vi "test_sampling.vi"() -> ()   [LabVIEW 2017]
uses:
  <vilib>/Analysis/2dsp.llb/1D Convolution (DBL).vi
  <vilib>/Analysis/NI_AALBase.lvlib
  <vilib>/Analysis/NI_AALPro.lvlib
panel:
  out "32비트 정수":i32
  out "FFT signal 3":waveform(dbl)(graph)
  out "FFT signal 2":waveform(dbl)(graph)
  out "크기 2":i32
  out "signal 2":waveform(dbl)(graph)
  in  "sampling time(sec)":dbl=0.5
  out "크기":i32
  out "Array":dbl[](array[numeric])
  out "FFT signal":waveform(dbl)(graph)
  out "signal":waveform(dbl)(graph)
  in  "Frequency(Hz)":dbl=614000.0
  in  "Amplitude(Vpeak)":dbl=1.0
  in  "Pulse length(sec)":dbl=0.5
  in  "Sampling frequency(Hz)":dbl=3000000.0
  in  "Delay time.A.1(sec)":dbl=0.5
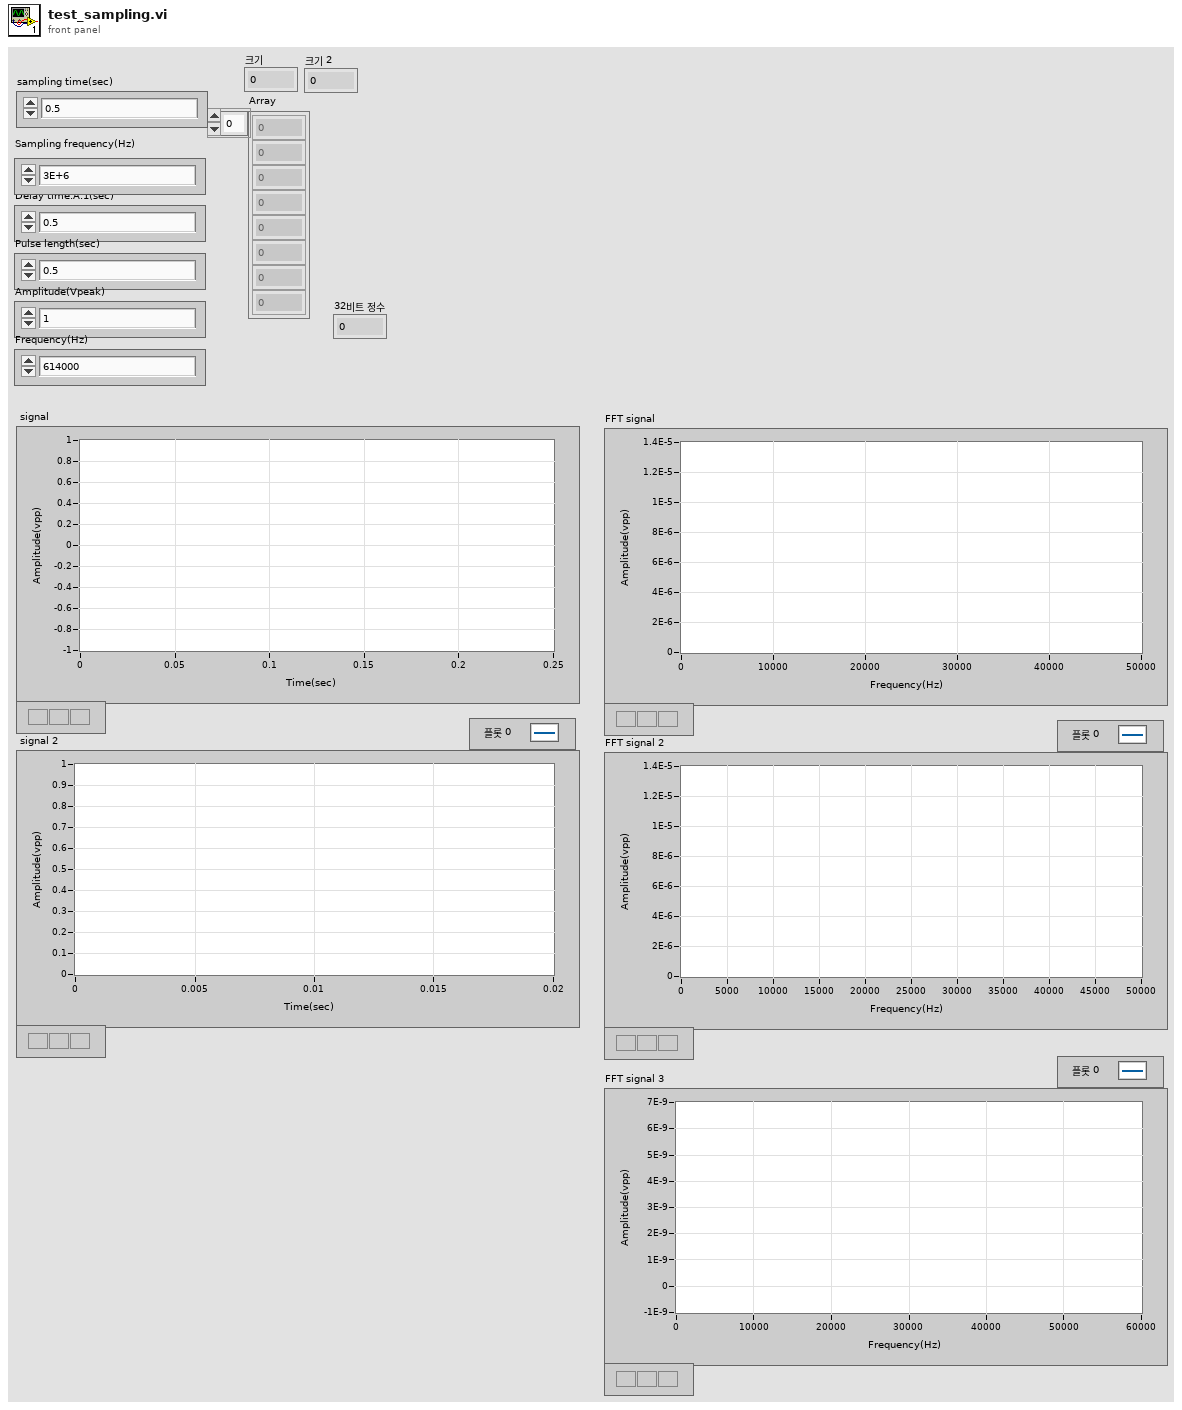
[diagram p1: front panel]
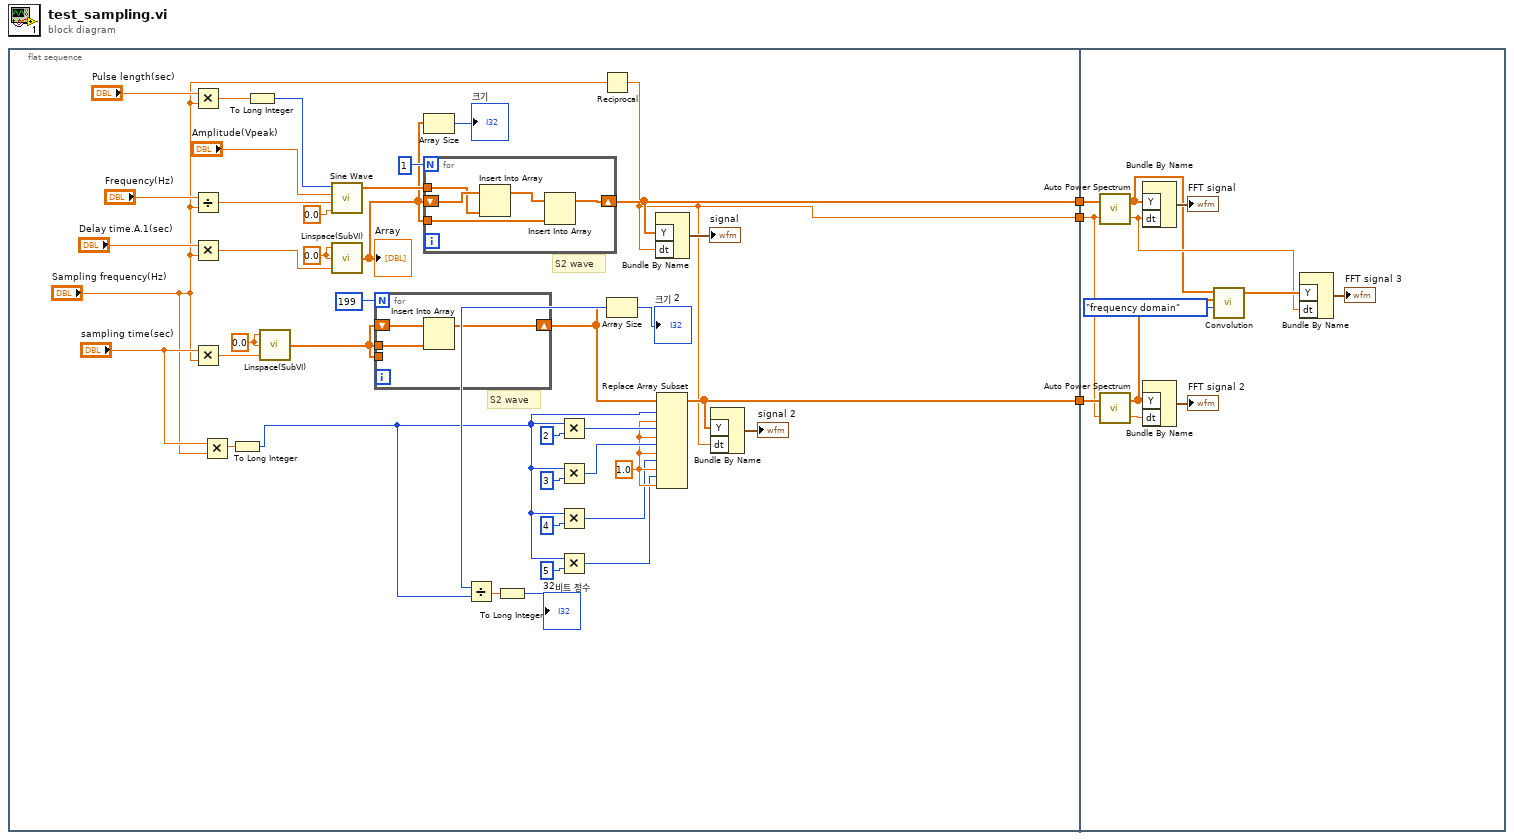
[diagram p0: block diagram]
diagram:
  n1 = flat-sequence {
    tunnel: [w30] -> w3
    tunnel: [w5] -> w2
    tunnel: [w19] -> w1
    tunnel: w3 -> [w63]
    tunnel: w2 -> [w58]
    tunnel: w1 -> [w59]
    frame #0 {
      w18 = 1.0 ("새 원소/부분배열")
      w27 = 0.0 ("Start")
      w36 = 0.0 ("Start")
      # "S2 wave"
      # "S2 wave"
      n2 = Multiply(x="Pulse length(sec)", y="Sampling frequency(Hz)") -> (x*y=w42:dbl)
      n3 = Divide(x="Frequency(Hz)", y="Sampling frequency(Hz)") -> (x/y=w38:dbl)
      n4 = Multiply(x="Delay time.A.1(sec)", y="Sampling frequency(Hz)") -> (x*y=w34:dbl)
      n5 = Multiply(x="sampling time(sec)", y="Sampling frequency(Hz)") -> (x*y=w26:dbl)
      n6 = Multiply(x="sampling time(sec)", y="Sampling frequency(Hz)") -> (x*y=w11:dbl)
      n7 = To Long Integer(number=w11) -> (32bit integer=w9:i32)
      n8 = To Long Integer(number=w42) -> (32bit integer=w41:i32)
      n9 = call "Linspace(SubVI).vi"("NumElements"=w26, "End"=w27, "Start"=w27) -> ("Array"=w7:dbl[])
      n10 = call <vilib>:"Sine Wave.vi"("samples"=w41, "amplitude"="Amplitude(Vpeak)", "frequency"=w38, "phase in"=0.0) -> ("sine wave"=w32:dbl[])  [unwired: 1 in, 2 out]
      n11 = call "Linspace(SubVI).vi"("NumElements"=w34, "End"=w36, "Start"=w36) -> ("Array"=w29:dbl[])
      "Array" <- w29
      n12 = for {
        N: 199 -> [_]
        shift-right: [w44] -> w6
        shift-left: w7 -> [w46]
        tunnel: w7 -> [w45]
        tunnel: w7 -> [_]
        n13 = Insert Into Array(array=w46, new element=w45) -> (w44:dbl[])  [unwired: 1 in]
      }
      n14 = Array Size(array=w29) -> (size(s)=→"크기":i32)
      n15 = for {
        N: 1 -> [_]
        shift-right: [w47] -> w30
        shift-left: w29 -> [w51]
        tunnel: w32 -> [w50]
        tunnel: w29 -> [w48]
        n16 = Insert Into Array(array=w51, new element=w50) -> (w49:dbl[])  [unwired: 1 in]
        n17 = Insert Into Array(array=w49, new element=w48) -> (w47:dbl[])  [unwired: 1 in]
      }
      n18 = Multiply(x=w9, y=2) -> (x*y=w22:i32)
      n19 = Multiply(x=w9, y=3) -> (x*y=w20:i32)
      n20 = Multiply(x=w9, y=4) -> (x*y=w16:i32)
      n21 = Multiply(x=w9, y=5) -> (x*y=w14:i32)
      n22 = Reciprocal(x="Sampling frequency(Hz)") -> (1/x=w5:dbl)
      n23 = Array Size(array=w6) -> (size(s)=w10:i32)
      "크기 2" <- w10
      n24 = Divide(x=w10, y=w9) -> (x/y=w8:dbl)
      n25 = To Long Integer(number=w8) -> (32bit integer=→"32비트 정수":i32)
      n26 = Bundle By Name("Y"=w30, "dt"=w5) -> (→"signal":waveform(dbl))  [unwired: 1 in]
      n27 = Replace Array Subset(array=w6, new element #1=w18, index #1=w9, new element #2=w18, index #2=w22, new element #3=w18, index #3=w20, new element #4=w18, index #4=w16, new element #5=w18, index #5=w14) -> (w19:dbl[])
      n28 = Bundle By Name("Y"=w19, "dt"=w5) -> (→"signal 2":waveform(dbl))  [unwired: 1 in]
    }
    frame #1 {
      n29 = call <vilib>:"Auto Power Spectrum.vi"("dt"=w58, "Signal (V)"=w63) -> ("df"=w55:dbl, "Power Spectrum (V^2 rms)"=w54:dbl[])
      n30 = call <vilib>:"Auto Power Spectrum.vi"("dt"=w58, "Signal (V)"=w59) -> ("df"=w60:dbl, "Power Spectrum (V^2 rms)"=w53:dbl[])
      n31 = Bundle By Name("Y"=w54, "dt"=w55) -> (→"FFT signal":waveform(dbl))  [unwired: 1 in]
      n32 = Bundle By Name("Y"=w53, "dt"=w60) -> (→"FFT signal 2":waveform(dbl))  [unwired: 1 in]
      n33 = call-poly <vilib>:"Convolution.vi"("algorithm"=enum32{"direct", "frequency domain"}."frequency domain", "Y"=w53, "X"=w54) -> ("X * Y"=w56:dbl[])  [unwired: 7 in, 1 out]
      n34 = Bundle By Name("Y"=w56, "dt"=w55) -> (→"FFT signal 3":waveform(dbl))  [unwired: 1 in]
    }
  }
